vi "Create Interpolated Color Palette.vi"(8 "Error In":errorcluster, 11 "Color Scale Points":cluster{"Value":dbl, "Color":u32}[](array[cluster])) -> (0 "Error Out":errorcluster, 3 "Interpolated Color Scale":u32[](array[colorbox]))   [LabVIEW 2021, in "Palette.lvlib"]
uses:
  Palette.lvlib
  <userlib>/_OpenG.lib/array/array.llb/Sort 1D Array (DBL)__ogtk.vi
  <userlib>/_OpenG.lib/array/array.llb/Reorder 1D Array2 (U32)__ogtk.vi
  <userlib>/_OpenG.lib/array/array.llb/openg_array.lvlib
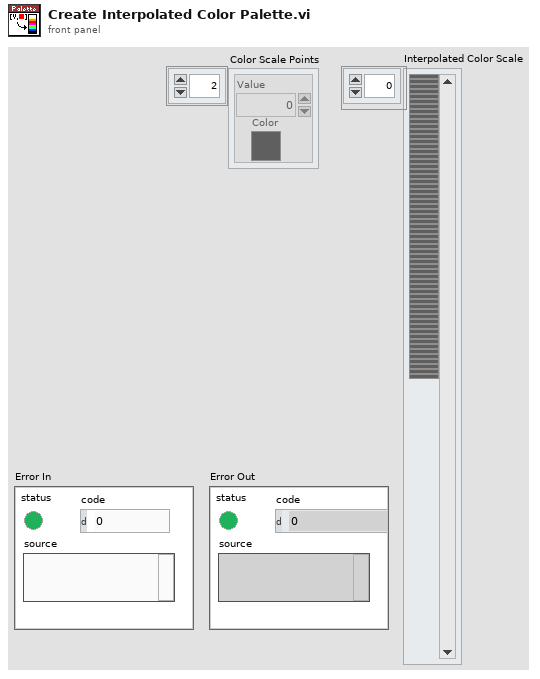
[diagram p1: front panel]
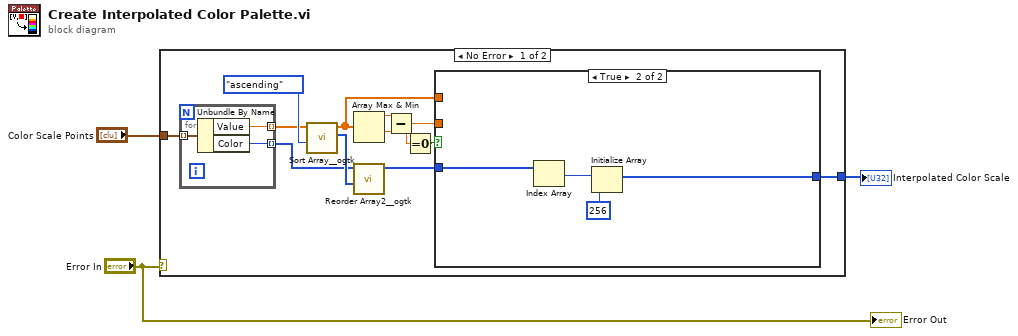
[diagram p0: block diagram]
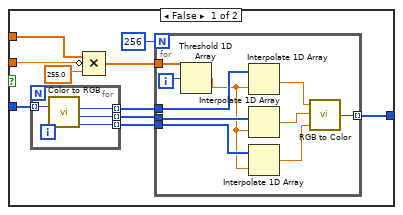
[diagram p2: hidden frame]
diagram:
  n1 = case shown="No Error" "Error In" {
    tunnel: "Color Scale Points" -> [w8 _]
    tunnel: [w6 _] -> w2
    frame No Error {
      n2 = for {
        tunnel: w8 -> [w46] mode=indexing
        tunnel: [w45] -> w9 mode=indexing
        tunnel: [w44] -> w11 mode=indexing
        n3 = Unbundle By Name(w46) -> ("Value"=w45:dbl, "Color"=w44:u32)
      }
      n4 = call-poly <userlib>:"Sort Array__ogtk.vi"("Order"=enum16{"ascending", "descending"}."ascending", "Array in"=w9) -> ("Sorted Pointers"=w12:i32[], "Sorted Array out"=w15:dbl[])  [unwired: 8 in]
      n5 = Array Max & Min(array=w15) -> (max value=w13:dbl, min value=w14:dbl)  [unwired: 2 out]
      n6 = call-poly <userlib>:"Reorder Array2__ogtk.vi"("indices"=w12, "array"=w11) -> ("reordered array"=w7:u32[])  [unwired: 9 in]
      n7 = Subtract(x=w13, y=w14) -> (x-y=w5:dbl)
      n8 = Equal To 0?(x=w5) -> (x = 0?=w4:bool)
      n9 = case shown="True" w4 {
        tunnel: w15 -> [w25 _]
        tunnel: w7 -> [w21 w43]
        tunnel: [w17 w40] -> w6
        tunnel: w5 -> [w16 _]
        frame False {
          n10 = for {
            tunnel: w21 -> [w29] mode=indexing
            tunnel: [w28] -> w20 mode=indexing
            tunnel: [w27] -> w19 mode=indexing
            tunnel: [w26] -> w18 mode=indexing
            n11 = call <vilib>:"Color to RGB.vi"("Color"=w29) -> ("R"=w28:u8, "G"=w27:u8, "B"=w26:u8)  [unwired: 1 out]
          }
          n12 = Compound Arithmetic op=MULTIPLY(w25, invert w16, 255.0 ("y")) -> (w22:dbl[])
          n13 = for {
            N: 256 -> [_]
            tunnel: w22 -> [w39]
            tunnel: w19 -> [w36]
            tunnel: w20 -> [w37]
            tunnel: w18 -> [w35]
            tunnel: [w30] -> w17 mode=indexing
            i -> [w38]
            n14 = Threshold 1D Array(2:w38, 3:w39) -> (0:w34:dbl)  [unwired: 1 in]
            n15 = Interpolate 1D Array(1:w34, 2:w37) -> (0:w33:dbl)
            n16 = Interpolate 1D Array(1:w34, 2:w36) -> (0:w32:dbl)
            n17 = Interpolate 1D Array(1:w34, 2:w35) -> (0:w31:dbl)
            n18 = call <vilib>:"RGB to Color.vi"("B"=w31, "G"=w32, "R"=w33) -> ("Color"=w30:u32)
          }
        }
        frame True {
          n19 = Index Array(array=w43) -> (element=w42:u32)  [unwired: 1 in]
          n20 = Initialize Array(w42, 256) -> (w40:u32[])
        }
      }
    }
    frame Error {
    }
  }
  "Interpolated Color Scale" <- w2
  "Error Out" <- "Error In"
